vi "Save All VI Data.vi"(8 "error in (no error)":errorcluster, 10 "Saved VI Data in":T1[](array[typedef]), 11 "New VI Data in":T1[](array[typedef])) -> (0 "error out":errorcluster, 2 "Saved VI Data out":T1[](array[typedef]), 3 "New VI Data out":T1[](array[typedef]))   [LabVIEW 2023, in "VI Properties Editor.lvlib"]
uses:
  VI Properties Editor.lvlib
  CTLs/VI Data.ctl
  <vilib>/picture/picture.llb/imagedata.ctl
  CTLs/VI Properties.ctl
  CTLs/Control Properties.ctl
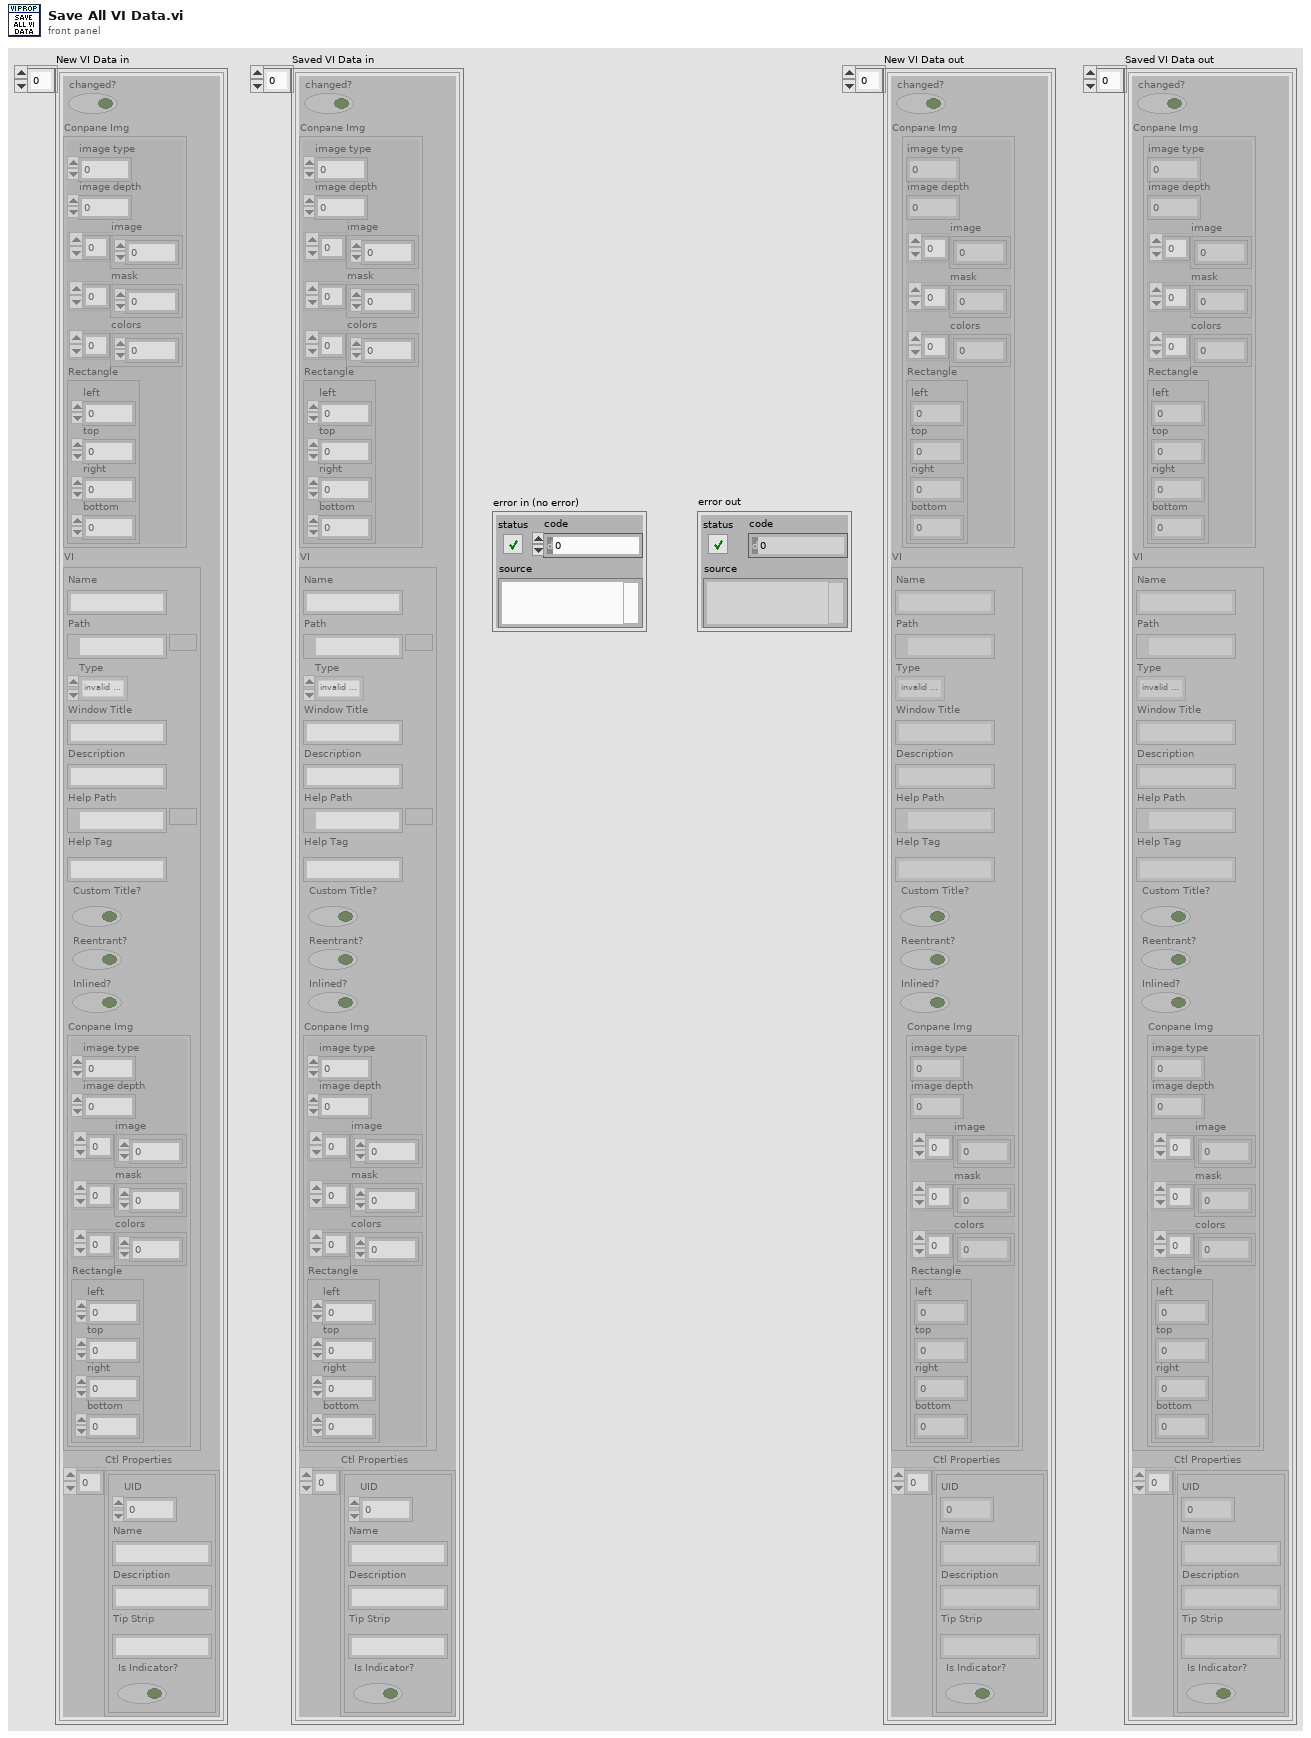
[diagram p1: front panel]
types:
  T1 = typedef "VI Properties Editor.lvlib/VI Data.ctl" = cluster{"changed?":bool, "Conpane Img":T2, "VI":T3, "Ctl Properties":T4[]}
  T2 = typedef "imagedata.ctl" = cluster{"image type":i32, "image depth":i32, "image":u8[], "mask":u8[], "colors":u32[], "Rectangle":cluster{"left":i16, "top":i16, "right":i16, "bottom":i16}}
  T3 = typedef "VI Properties Editor.lvlib/VI Properties.ctl" = cluster{"Name":string, "Path":path, "Type":enum32{"invalid VI type", "Standard VI", "Control VI", "Global VI", "Polymorphic VI", "Configuration VI", "SubSystem", "Facade VI", "Method VI", "Statechart Diagram VI"}, "Window Title":string, "Description":string, "Help Path":path, "Help Tag":string, "Custom Title?":bool, "Reentrant?":bool, "Inlined?":bool, "Conpane Img":T2}
  T4 = typedef "VI Properties Editor.lvlib/Control Properties.ctl" = cluster{"UID":i32, "Name":string, "Description":string, "Tip Strip":string, "Is Indicator?":bool}
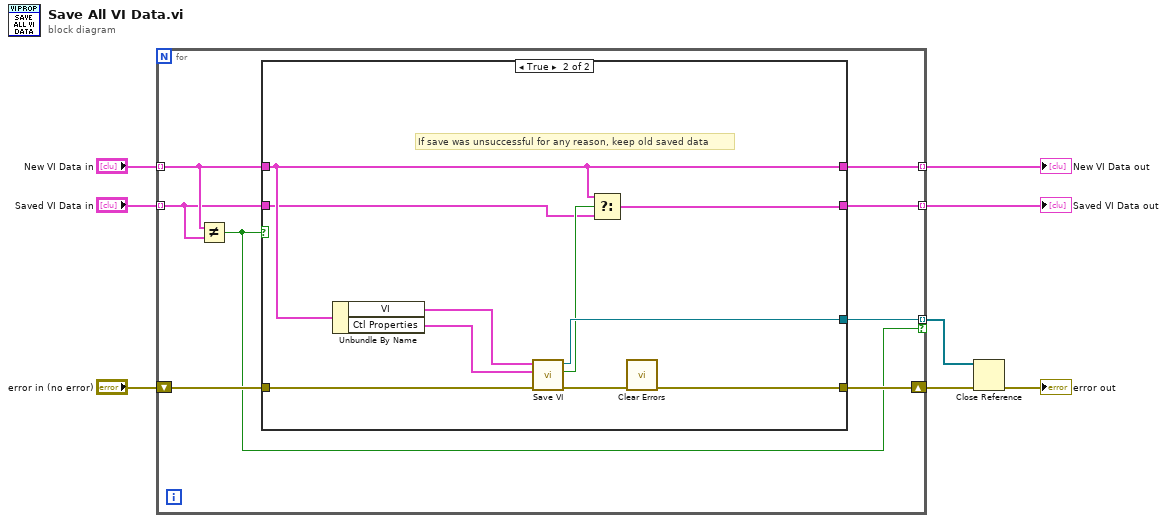
[diagram p0: block diagram]
diagram:
  n1 = for {
    shift-right: [w14] -> w5
    shift-left: "error in (no error)" -> [w16]
    tunnel: "New VI Data in" -> [w13] mode=indexing
    tunnel: [w15] -> w4 mode=indexing if=w11
    tunnel: [w12] -> w7 mode=indexing
    tunnel: "Saved VI Data in" -> [w10] mode=indexing
    tunnel: [w9] -> w1 mode=indexing
    n2 = Not Equal?(x=w13, y=w10) -> (x != y?=w11:bool)
    n3 = case shown="True" w11 {
      tunnel: w16 -> [w17 w29]
      tunnel: [_ w28] -> w15
      tunnel: [w17 w27] -> w14
      tunnel: w13 -> [w19 w22]
      tunnel: [w19 w22] -> w12
      tunnel: w10 -> [w18 w21]
      tunnel: [w18 w20] -> w9
      frame False {
      }
      frame True {
        # "If save was unsuccessful for any reason, keep old saved data"
        n4 = Unbundle By Name(w22) -> ("VI"=w24:T3, "Ctl Properties"=w25:T4[])
        n5 = call "Save VI.vi"("error in (no error)"=w29, "Ctl Properties"=w25, "VI Properties"=w24) -> ("error out"=w26:errorcluster, "Saved?"=w23:bool, "VI out"=w28:refnum<vi>)  [unwired: 6 in]
        n6 = Select(t=w22, s=w23, f=w21) -> (s? t:f=w20:T1)
        n7 = call <vilib>:"Clear Errors.vi"("error in (no error)"=w26) -> ("error out"=w27:errorcluster)  [unwired: 5 in, 1 out]
      }
    }
  }
  "New VI Data out" <- w7
  "Saved VI Data out" <- w1
  n8 = Close Reference(reference=w4, error in (no error)=w5) -> (error out=→"error out":errorcluster)
